vi "Export Data tsv.vi"(5 "Wavelengths":dbl[](array[numeric]), 6 "Comments":string="Comment Thread", 7 "Channel Names":string[](array[string]), 8 "error in (no error)":errorcluster, 9 "Raw Data":dbl[][](array[numeric]), 10 "Processed Data":dbl[](array[numeric]), 11 "File Name":path) -> (0 "error out":errorcluster)   [LabVIEW 2023]
doc: "Writes Arrays to individual sheets in one Excel Workbook. The same Comments box and Channel Names are written to each sheet.\n\nData passed to this should be arranged in columns."
uses:
  File IO/Data File Header Constants.vi
  File IO/File IO.lvclass
panel:
  out "spreadsheet string":string
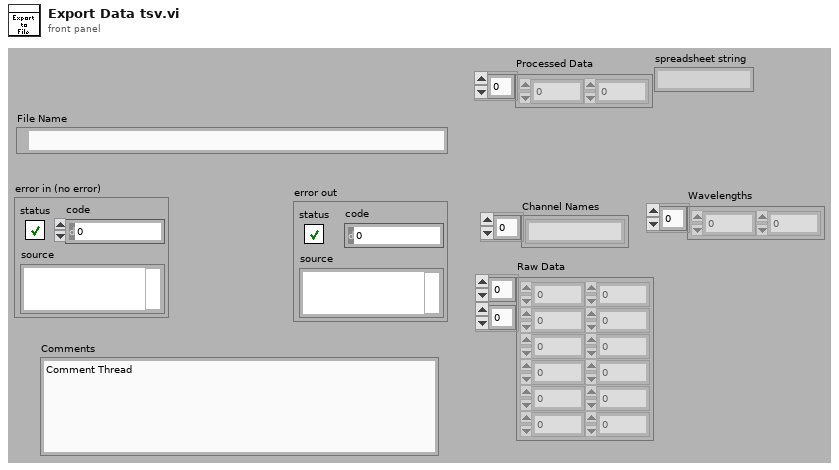
[diagram p1: front panel]
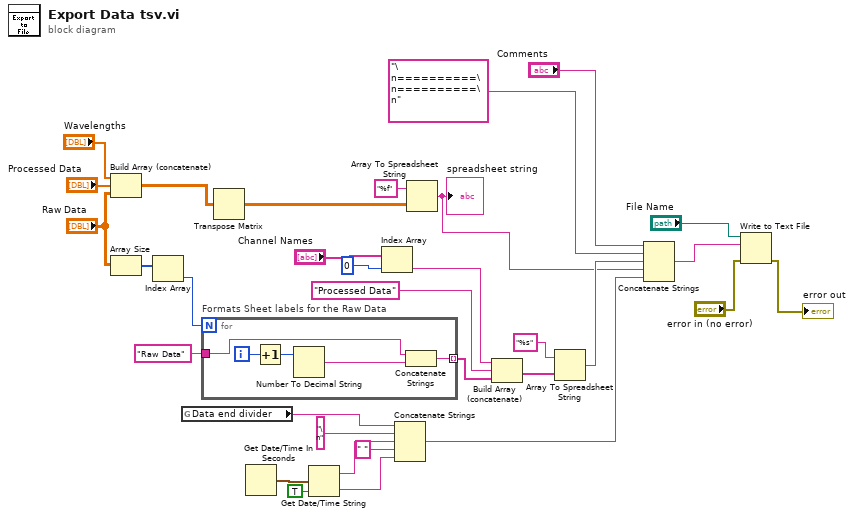
[diagram p0: block diagram]
diagram:
  n1 = Build Array (concatenate)("Wavelengths", "Processed Data", "Raw Data") -> (w22:dbl[][])
  n2 = Array Size(array="Raw Data") -> (size(s)=w32:i32[])
  n3 = Index Array(array=w32) -> (element=w31:i32)  [unwired: 1 in]
  n4 = global read "Data File Header Constants.vi" "Data end divider"() -> (w5:string)
  n5 = for "Formats Sheet labels for the Raw Data" {
    N: w31 -> [_]
    tunnel: "Raw Data" -> [w37]
    tunnel: [w35] -> w26 mode=indexing
    i -> [w34]
    n6 = Increment(x=w34) -> (x+1=w33:i32)
    n7 = Number To Decimal String(number=w33) -> (decimal integer string=w36:string)  [unwired: 1 in]
    n8 = Concatenate Strings(w37, w36) -> (w35:string)
  }
  n9 = Transpose Matrix(1:w22) -> (0:w21:dbl[][])
  n10 = Get Date/Time In Seconds() -> (seconds since 1Jan1904=w10:timestamp)
  n11 = Get Date/Time String(seconds (now)=w10, want seconds? (F)=TRUE) -> (date string=w9:string, time string=w3:string)  [unwired: 1 in]
  n12 = Index Array(array="Channel Names", index=0) -> (element=w12:string)
  n13 = Concatenate Strings(w5, "\n" ("string"), w9, " " ("string"), w3) -> (w8:string)
  n14 = Array To Spreadsheet String(array=w21, 3:"%f" ("format string")) -> (spreadsheet string=w17:string)  [unwired: 1 in]
  "spreadsheet string" <- w17
  n15 = Build Array (concatenate)(w12, "Processed Data", w26) -> (w19:string[])
  n16 = Array To Spreadsheet String(array=w19, 3:"%s" ("format string")) -> (spreadsheet string=w18:string)  [unwired: 1 in]
  n17 = Concatenate Strings("Comments", "\n==========\n==========\n" ("string"), w18, w17, w8) -> (w16:string)
  n18 = Write to Text File(file (use dialog)="File Name", text=w16, error in="error in (no error)") -> (error out=→"error out":errorcluster)  [unwired: 1 in, 2 out]
